vi "20220127-main.vi"   [LabVIEW 2019]
uses:
  subVI/move/position cluster.ctl
  subVI/move/move array.ctl
  <vilib>/myRIO/Instrument Drivers/Utilities/Utilities.lvlib
types:
  T1 = typedef "move array.ctl" = cluster{"X":dbl, "Y":dbl}[]
  T2 = typedef "position cluster.ctl" = cluster{"X":dbl, "Y":dbl, "Angle":dbl}
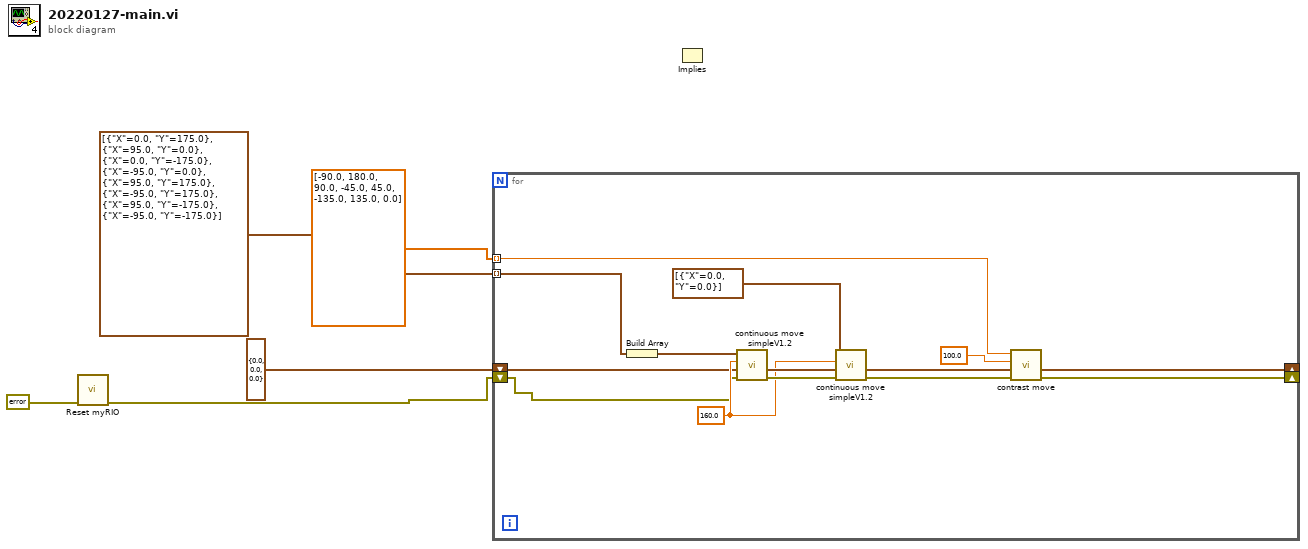
[diagram p0: block diagram]
diagram:
  n1 = call <vilib>:"Reset myRIO.vi"("error in (no error)"=errorcluster {"status"=FALSE, "code"=0, "source"=""} ("error constant")) -> ("error out"=w1:errorcluster)  [unwired: 10 in]
  n2 = for {
    shift-right: [w16] -> _
    shift-left: T2 {"X"=0.0, "Y"=0.0, "Angle"=0.0} ("Position out") -> [w12]
    tunnel: T1 [{"X"=0.0, "Y"=175.0}, {"X"=95.0, "Y"=0.0}, {"X"=0.0, "Y"=-175.0}, {"X"=-95.0, "Y"=0.0}, {"X"=95.0, "Y"=175.0}, {"X"=-95.0, "Y"=175.0}, {"X"=95.0, "Y"=-175.0}, {"X"=-95.0, "Y"=-175.0}] ("Array") -> [w10] mode=indexing
    tunnel: dbl[] [-90.0, 180.0, 90.0, -45.0, 45.0, -135.0, 135.0, 0.0] ("Target degree") -> [w8] mode=indexing
    shift-right: [w7] -> _
    shift-left: w1 -> [w6]
    w13 = 160.0 ("Speed")
    n3 = Build Array(w10) -> (w11:cluster{"X":dbl, "Y":dbl}[])
    n4 = call "continuous move simpleV1.2.vi"("error in (no error)"=w6, "Position"=w12, "Speed"=w13, "Array"=w11) -> ("error out"=w14:errorcluster, "Position out"=w15:T2)  [unwired: 6 in]
    n5 = call "continuous move simpleV1.2.vi"("error in (no error)"=w14, "Position"=w15, "Speed"=w13, "Array"=T1 [{"X"=0.0, "Y"=0.0}]) -> ("error out"=w19:errorcluster, "Position out"=w18:T2)  [unwired: 6 in]
    n6 = call "contrast move.vi"("error in (no error)"=w19, "Position in"=w18, "speed"=100.0, "Target degree"=w8) -> ("error out"=w7:errorcluster, "Position out"=w16:T2)  [unwired: 6 in]
  }
  n7 = Implies() -> ()  [unwired: 2 in, 1 out]
